vi "GFBuildTriggerWaveForm.vi"(0 "Trigger Data Input":T4, 1 "Selected Board":T1, 2 "TS Ref Shot":bool, 3 "error in":errorcluster, 4 "task in":refnum<k21>="USB-MagAndTrigFire") -> (5 "Digital Waveform Graph":digitalwaveform[](graph), 6 "error out":errorcluster)   [LabVIEW 2009]
doc: "Magnet timing pulses should be input relative to fast fire pulse, at most 2 s behind (-2 to 0 s)"
uses:
  Signal Clustering/Ctrl_Signal.ctl
  Signal Clustering/Ctrl_Signal_Map.ctl
  Program Files (x86)/National Instruments/LabVIEW 2009/resource/objmgr/daqmx.rc
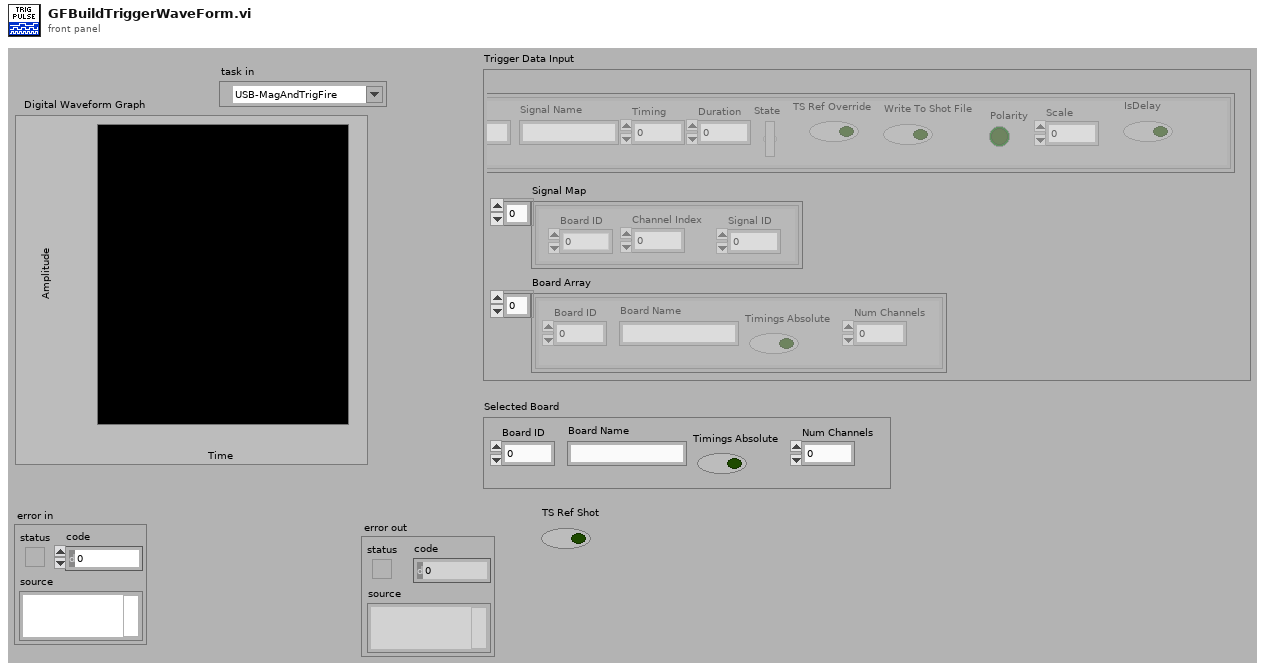
[diagram p1: front panel]
types:
  T1 = cluster{"Board ID":dbl, "Board Name":string, "Timings Absolute":bool, "Num Channels":dbl}
  T2 = typedef "Ctrl_Signal.ctl" = cluster{"Signal Name":string, "Timing":dbl, "Duration":dbl, "State":bool, "TS Ref Override":bool, "Write To Shot File":bool, "Polarity":bool, "Signal ID":dbl, "Scale":dbl, "IsDelay":bool}
  T3 = typedef "Ctrl_Signal_Map.ctl" = cluster{"Channel Index":dbl, "Board ID":dbl, "Signal ID":dbl}
  T4 = cluster{"Signal Array":T2[], "Signal Map":T3[], "Board Array":cluster{"Board ID":dbl, "Board Name":string, "Timings Absolute":bool, "Num Channels":dbl}[]}
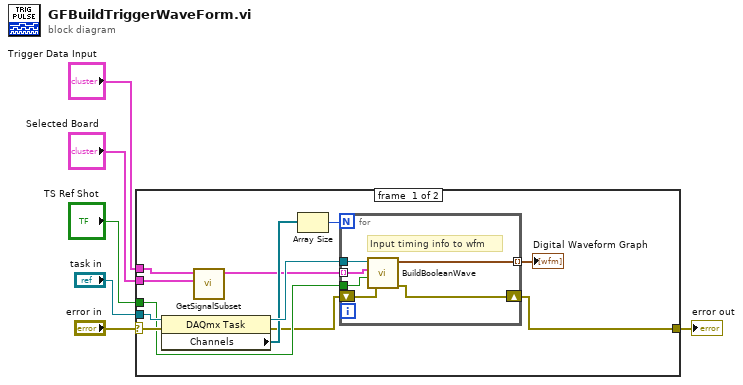
[diagram p0: block diagram]
diagram:
  n1 = case shown="No Error" "error in" {
    selector: "error in" -> [w17 w25]
    tunnel: "task in" -> [w18 _]
    tunnel: [w7 w25] -> w4
    tunnel: "Selected Board" -> [w11 _]
    tunnel: "Trigger Data Input" -> [w12 _]
    tunnel: "TS Ref Shot" -> [w10 _]
    frame #0 {
      n2 = property class="DAQmx Task"(reference=w18, error in=w17) -> (reference out=w14:refnum<k21>, error out=w8:errorcluster, "Channels"=w13:refnum<k21>[])
      n3 = call "GetSignalSubset.vi"("Selected Board"=w11, "Trigger Data Input"=w12) -> ("Signal Subset"=w9:T2[])  [unwired: 9 in]
      n4 = Array Size(array=w13) -> (size(s)=w15:i32)
      n5 = for {
        N: w15 -> [_]
        tunnel: w14 -> [w24]
        tunnel: [w23] -> w16 mode=indexing
        tunnel: w9 -> [w22] mode=indexing
        tunnel: w10 -> [w21]
        shift-right: [w19] -> w7
        shift-left: w8 -> [w20]
        # "Input timing info to wfm"
        n6 = call "BuildBooleanWave.vi"("DAQmx Global Channel"=w24, "Ctrl_Signal"=w22, "TS RefShot"=w21, "error in (no error)"=w20) -> ("waveform out"=w23:digitalwaveform, "error out"=w19:errorcluster)  [unwired: 4 in]
      }
      "Digital Waveform Graph" <- w16
    }
    frame #1 {
    }
  }
  "error out" <- w4
